vi "UI Direct Message.vi"(8 "error in (no error)":errorcluster, 10 "Message Cluster":T1, 11 "Chat Room Model in":refnum<class "Chat Room Model.lvclass">) -> (0 "error out":errorcluster, 3 "Chat Room Model out":refnum<class "Chat Room Model.lvclass">)   [LabVIEW 2020, in "Chat Room Model.lvlib" / "Chat Room Model.lvclass"]
uses:
  Chat Room Model.lvclass
  Chat Room Model.lvclass/Chat Room Model.ctl
  Application Control/Message.ctl
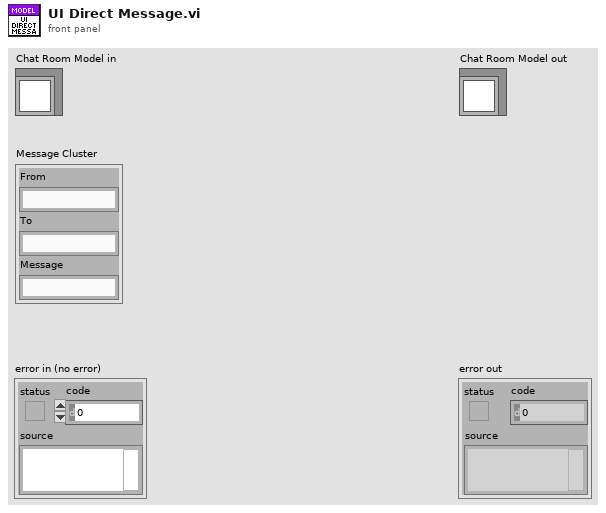
[diagram p1: front panel]
types:
  T1 = typedef "Message.ctl" = cluster{"From":string, "To":string, "Message":string}
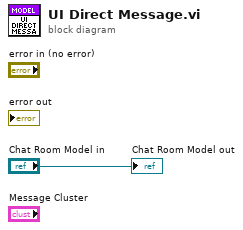
[diagram p0: block diagram]
diagram:
  "Chat Room Model out" <- "Chat Room Model in"
